vi "Get Cal Director.vi"(6 "기술책임자 참조":refnum<vi>, 8 "에러 입력(에러 없음)":errorcluster, 10 "교정정보 in":T1, 11 "참조 번호 입력":T2) -> (0 "에러 출력":errorcluster, 1 "기책 사번":string, 2 "교정정보 out":T1, 3 "참조 번호 출력":T2)   [LabVIEW 2020]
uses:
  Controls/Clst_Cal Info Global.ctl
  <vilib>/addons/database/Connection.llb/Conn ObjectReference.ctl
  Controls/Cmd_Read Query.ctl
  Controls/Clst_Query Info.ctl
  Public/Polymorph/Array Dedup_1D Str.vi
  <vilib>/addons/database/NI_Database_API.lvlib
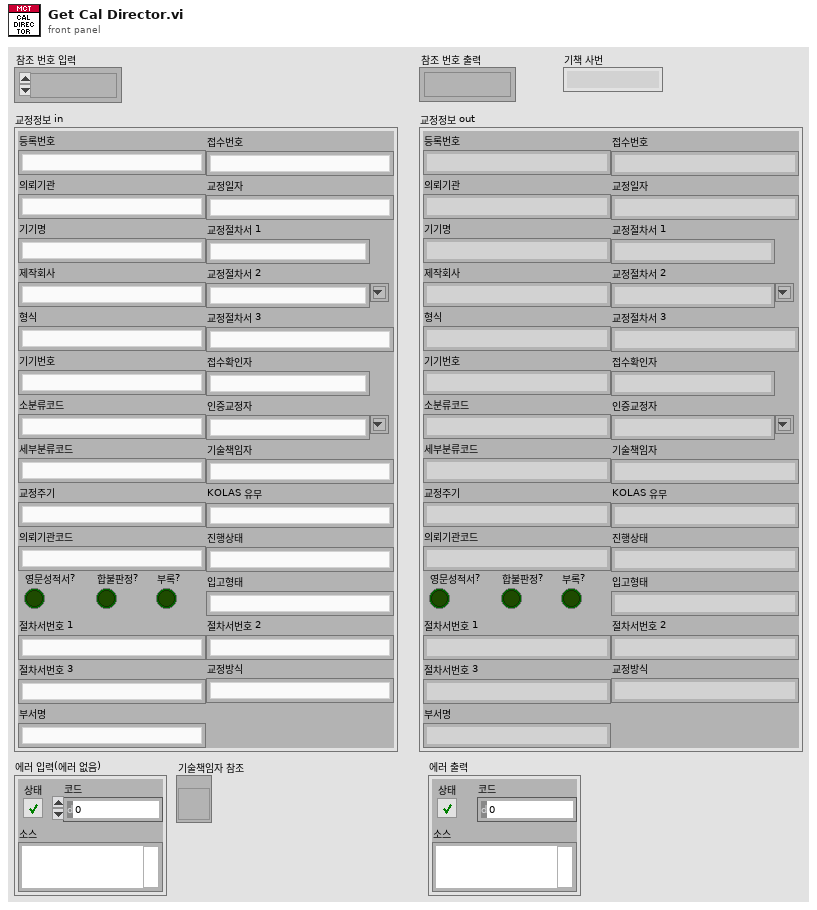
[diagram p1: front panel]
types:
  T1 = typedef "Clst_Cal Info Global.ctl" = cluster{"등록번호":string, "의뢰기관":string, "기기명":string, "제작회사":string, "형식":string, "기기번호":string, "소분류코드":string, "세부분류코드":string, "교정주기":string, "접수번호":string, "교정일자":string, "교정절차서 1":string, "교정절차서 2":string, "교정절차서 3":string, "접수확인자":string, "인증교정자":string, "기술책임자":string, "KOLAS 유무":string, "진행상태":string, "의뢰기관코드":string, "입고형태":string, "영문성적서?":bool, "합불판정?":bool, "부록?":bool, "절차서번호 1":string, "절차서번호 2":string, "절차서번호 3":string, "교정방식":string, "부서명":string}
  T2 = typedef "NI_Database_API.lvlib/Conn ObjectReference.ctl" = refnum<k1>
  T3 = typedef "Clst_Query Info.ctl" = cluster{"사번":string, "등록번호":string, "업체명":string, "세부분류코드":string, "형식":string, "기기번호":string, "FUNC":string, "FUNC_EXT":string, "옵션":string, "추가문자열":string, "일자":string, "배열 1":string[], "배열 2":string[], "항목명":string, "문자열":string, "이름":string}
  T4 = typedef "Cmd_Read Query.ctl" = enum16{"교정자 이름 얻기", "인증교정자 얻기", "기술책임자 얻기", "기책부책 얻기", "등록번호 얻기", "등록정보 얻기", "업체정보 얻기", "교정일자(CAMAS) 얻기", "교정일자(CALSTD) 얻기", "교정환경 얻기", "교정절차서 목록 얻기", "교정절차서명 얻기", "교정절차 목록얻기", "교정절차 얻기", "PROC 교정절차 얻기", "PROC SPEC 얻기", "교정절차(Func별) 얻기", "교정절차(Func_ext별) 얻기", "기관코드 얻기", "교정기능(세부분류) 얻기", "교정기능(모델) 얻기", "교정기능 목록 얻기", "교정기능 명칭 얻기", "교정기능 항목명칭 얻기", "DB (사용기준기) 얻기", "DB (기준기이름) 얻기", "DB (기준기이름목록) 얻기", "DB (기준기목록) 얻기", "DB (기준기값) 얻기", "DB (CMC) 얻기", "DB (FUNC) 얻기", "DB (CALNAME) 얻기", "DB (STDNAME) 얻기", "DB (SPEC) 얻기", "모델(항목전체) 얻기", "모델(최대범위) 얻기", "모델(최소범위) 얻기", "모델(최대최소) 얻기", "모델(범위조건) 얻기", "모델(등록요청) 얻기", "모델(형식별) 얻기", "모델(조건별) 얻기", "모델(모델검색) 얻기", "세부분류 목록 얻기", "기준기등록리스트 얻기", "STD Cal Date Check", "DB등록일자 얻기", "적용항목 얻기", "기타정보 얻기", "기준기요청 얻기", "서버버전 얻기"}
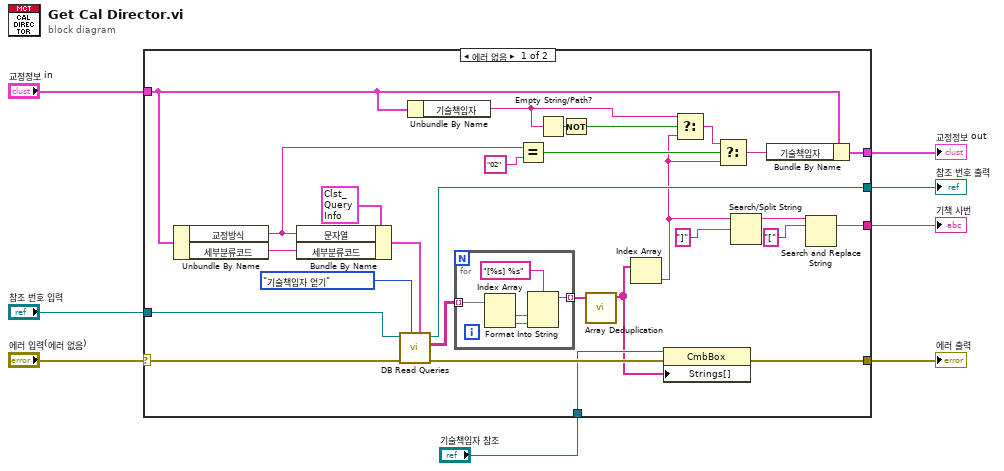
[diagram p0: block diagram]
diagram:
  n1 = case shown="에러 없음" "에러 입력(에러 없음)" {
    selector: "에러 입력(에러 없음)" -> [w29 w44]
    tunnel: [w32 w42] -> w8
    tunnel: "참조 번호 입력" -> [w31 w42]
    tunnel: [w27 w44] -> w6
    tunnel: [w21 _] -> w5
    tunnel: "교정정보 in" -> [w16 w43]
    tunnel: [w30 w43] -> w3
    tunnel: "기술책임자 참조" -> [w26 _]
    frame No Error {
      n2 = Unbundle By Name(w16) -> ("교정방식"=w18:string, "세부분류코드"=w35:string)
      n3 = Bundle By Name(cluster=T3 {"사번"="", "등록번호"="", "업체명"="", "세부분류코드"="", "형식"="", "기기번호"="", "FUNC"="", "FUNC_EXT"="", "옵션"="", "추가문자열"="", "일자"="", "배열 1"=[], "배열 2"=[], "항목명"="", "문자열"="", "이름"=""} ("Query info"), "문자열"=w18, "세부분류코드"=w35) -> (w36:T3)
      n4 = call "DB Read Queries.vi"("Query info"=w36, "Query Command"=Cmd_Read_Query."기술책임자 얻기", "에러 입력(에러 없음)"=w29, "참조 번호 입력"=w31) -> ("에러 출력"=w28:errorcluster, "Data"=w25:string[][], "참조 번호 출력"=w32:T2)  [unwired: 3 in, 2 out]
      n5 = Unbundle By Name(w16) -> ("기술책임자"=w13:string)
      n6 = for {
        tunnel: w25 -> [w40] mode=indexing
        tunnel: [w37] -> w24 mode=indexing
        n7 = Index Array(array=w40) -> (element #1=w39:string, element #2=w38:string)  [unwired: 2 in]
        n8 = Format Into String(format string="[%s] %s" ("포맷 문자열"), w39, w38) -> (resulting string=w37:string)  [unwired: 2 in, 1 out]
      }
      n9 = Equal?(x=w18, y="02") -> (x = y?=w15:bool)
      n10 = Empty String/Path?(string/path=w13) -> (empty?=w14:bool)
      n11 = Not(x=w14) -> (.not. x?=w9:bool)
      n12 = call-poly "Array Deduplication.vi"("배열 in"=w24) -> ("배열 out"=w23:string[])  [unwired: 9 in, 1 out]
      n13 = Index Array(array=w23) -> (element=w12:string)  [unwired: 1 in]
      n14 = property class="CmbBox"(reference=w26, error in=w28, "Strings[]"=w23) -> (error out=w27:errorcluster)  [unwired: 1 out]
      n15 = Select(t=w13, s=w9, f=w12) -> (s? t:f=w11:string)
      n16 = Select(t=w11, s=w15, f=w12) -> (s? t:f=w10:string)
      n17 = Search/Split String(string=w12, search string/char (-)="]" ("검색 문자열/문자 (-)")) -> (substring before match=w20:string)  [unwired: 1 in, 2 out]
      n18 = Bundle By Name(cluster=w16, "기술책임자"=w10) -> (w30:T1)
      n19 = Search and Replace String(input string=w20, search string="[" ("검색 문자열")) -> (result string=w21:string)  [unwired: 6 in, 3 out]
    }
    frame Error {
    }
  }
  "기책 사번" <- w5
  "참조 번호 출력" <- w8
  "에러 출력" <- w6
  "교정정보 out" <- w3
